vi "RunVIRefnum.vi"(8 "Error In":errorcluster, 9 "Settings":T1, 10 "JSON Input":string, 11 "VI Refnum In":refnum<vi>) -> (0 "Error Out":errorcluster, 2 "JSON Output":string, 3 "VI Refnum Out":refnum<vi>)   [LabVIEW 2019, in "LabJSON.lvlib"]
doc: "Take JSON as input, run the VI, and return the output as JSON"
uses:
  LabJSON.lvlib
  Typedefs/Settings.ctl
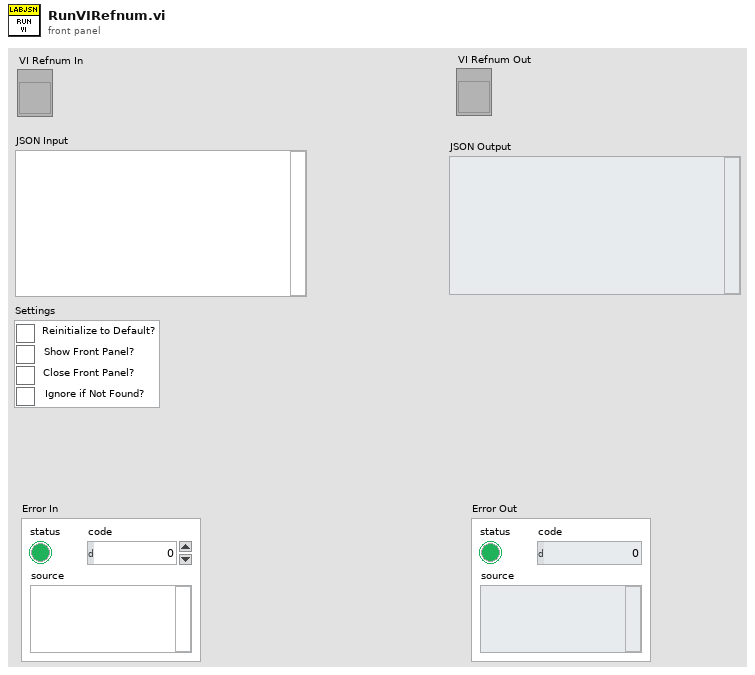
[diagram p1: front panel]
types:
  T1 = typedef "LabJSON.lvlib/Settings.ctl" = cluster{"Reinitialize to Default?":bool, "Show Front Panel?":bool, "Close Front Panel?":bool, "Ignore if Not Found?":bool}
  T2 = enum32{"Invalid", "Standard", "Closed", "Hidden", "Minimized", "Maximized"}
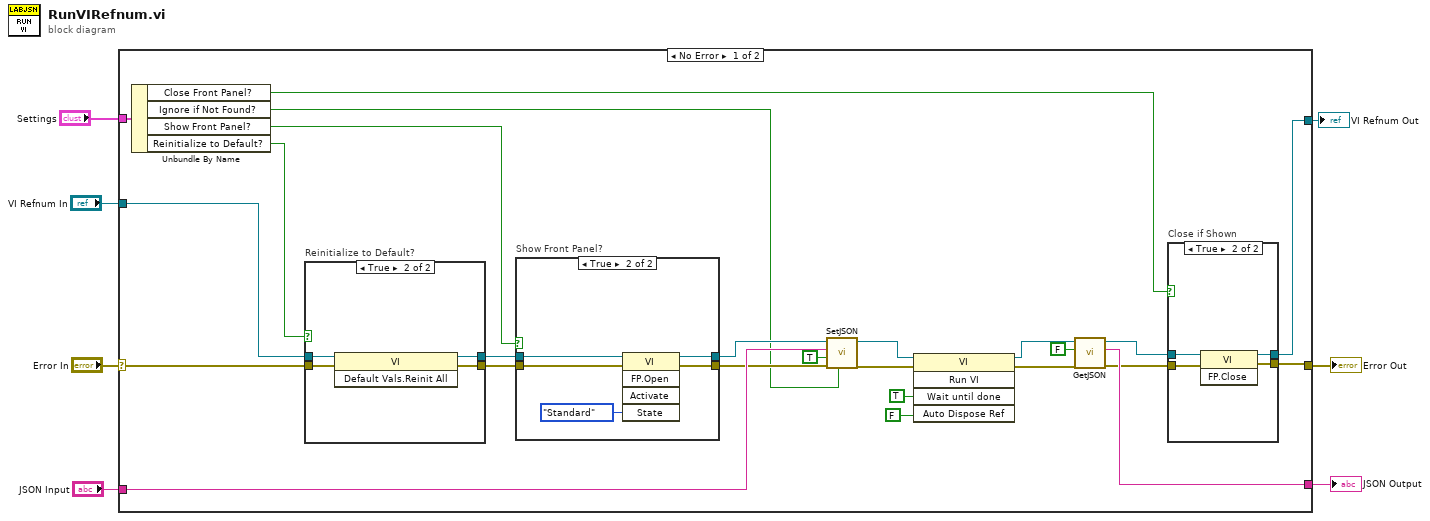
[diagram p0: block diagram]
diagram:
  n1 = case shown="No Error" "Error In" {
    selector: "Error In" -> [w19 w53]
    tunnel: [w20 w53] -> w6
    tunnel: "JSON Input" -> [w32 _]
    tunnel: "VI Refnum In" -> [w23 w52]
    tunnel: [w31 _] -> w3
    tunnel: [w12 w52] -> w2
    tunnel: "Settings" -> [w24 _]
    frame No Error {
      n2 = Unbundle By Name(w24) -> ("Close Front Panel?"=w11:bool, "Ignore if Not Found?"=w8:bool, "Show Front Panel?"=w14:bool, "Reinitialize to Default?"=w16:bool)
      n3 = case "Reinitialize to Default?" shown="True" w16 {
        tunnel: w23 -> [w47 w51]
        tunnel: [w47 w50] -> w22
        tunnel: w19 -> [w46 w49]
        tunnel: [w46 w48] -> w18
        frame False {
        }
        frame True {
          n4 = invoke class="VI" method="Default Vals.Reinit All"(reference=w51, error in=w49) -> (reference out=w50:refnum<vi>, error out=w48:errorcluster)  [unwired: 1 in, 1 out]
        }
      }
      n5 = case "Show Front Panel?" shown="True" w14 {
        tunnel: w22 -> [w40 w45]
        tunnel: w18 -> [w39 w44]
        tunnel: [w39 w43] -> w17
        tunnel: [w40 w41] -> w15
        frame False {
        }
        frame True {
          n6 = invoke class="VI" method="FP.Open"(reference=w45, error in=w44, "State"=T2."Standard") -> (reference out=w41:refnum<vi>, error out=w43:errorcluster)  [unwired: 2 in, 3 out]
        }
      }
      n7 = call "SetJSON.vi"("Ignore if Not Found?"=w8, "Error In"=w17, "Controls?"=TRUE, "JSON Input"=w32, "VI Refnum In"=w15) -> ("Error Out"=w30:errorcluster, "VI Refnum Out"=w29:refnum<vi>)  [unwired: 5 in]
      n8 = invoke class="VI" method="Run VI"(reference=w29, error in=w30, "Wait until done"=TRUE ("Wait Until Done"), "Auto Dispose Ref"=FALSE ("Auto Dispose Reference")) -> (reference out=w26:refnum<vi>, error out=w27:errorcluster)  [unwired: 1 in, 3 out]
      n9 = call "GetJSON.vi"("Error In"=w27, "Controls?"=FALSE, "VI Refnum In"=w26) -> ("Error Out"=w21:errorcluster, "JSON Out"=w31:string, "VI Refnum Out"=w13:refnum<vi>)  [unwired: 6 in]
      n10 = case "Close if Shown" shown="True" w11 {
        tunnel: w21 -> [w33 w38]
        tunnel: [w33 w37] -> w20
        tunnel: w13 -> [w34 w36]
        tunnel: [w34 w35] -> w12
        frame False {
        }
        frame True {
          n11 = invoke class="VI" method="FP.Close"(reference=w36, error in=w38) -> (reference out=w35:refnum<vi>, error out=w37:errorcluster)  [unwired: 1 in, 1 out]
        }
      }
    }
    frame Error {
    }
  }
  "JSON Output" <- w3
  "Error Out" <- w6
  "VI Refnum Out" <- w2
